vi "Get Ingredients.vi"(8 "error in (no error)":errorcluster, 11 "Metal Case in":refnum<class "Metal Case.lvclass">) -> (0 "error out":errorcluster, 2 "Ingredients":T1[](array[typedef]), 3 "Metal Case out":refnum<class "Metal Case.lvclass">)   [LabVIEW 2020, in "Metal Case.lvclass"]
uses:
  Metal Case.lvclass
  Item/Ingredient.ctl
  Item/Item.lvclass
  Metal/Metal.lvclass
  C:/dev/LabVIEW/Good Company Calc/Item/Item.lvclass
  Plastic/Plastic.lvclass
  Simple Case/Simple Case.lvclass
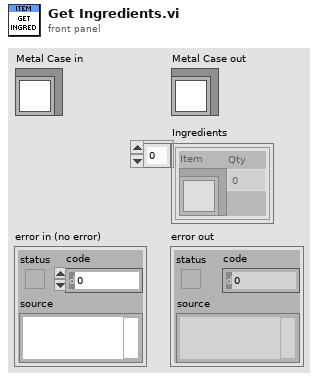
[diagram p1: front panel]
types:
  T1 = typedef "Item.lvclass/Ingredient.ctl" = cluster{"Item":refnum<class "Item.lvclass">, "Qty":dbl}
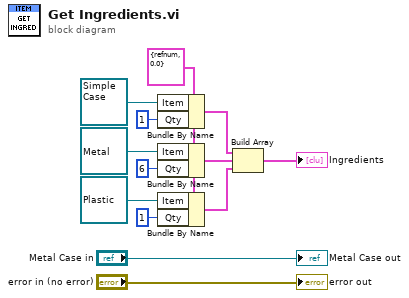
[diagram p0: block diagram]
diagram:
  w6 = T1 {"Item"=refnum, "Qty"=0.0} ("Ingredient")
  n1 = Bundle By Name(cluster=w6, "Item"=refnum<class "Simple Case.lvclass"> refnum ("Simple Case.lvclass"), "Qty"=1) -> (w3:T1)
  n2 = Bundle By Name(cluster=w6, "Item"=refnum<class "Metal.lvclass"> refnum ("Metal.lvclass"), "Qty"=6) -> (w5:T1)
  n3 = Bundle By Name(cluster=w6, "Item"=refnum<class "Plastic.lvclass"> refnum ("Plastic.lvclass"), "Qty"=1) -> (w4:T1)
  n4 = Build Array(w3, w5, w4) -> (→"Ingredients":T1[])
  "error out" <- "error in (no error)"
  "Metal Case out" <- "Metal Case in"
